vi "HW XML Rx - Write.vi"(0 "String (in)":string, 2 "Selected Channels":i32[](array[numeric]), 7 "Parameter Array":T1[](array[typedef])) -> (4 "String (out)":string)   [LabVIEW 2017]
uses:
  Controls/Database_Array.ctl
  Controls/Encoding.ctl
  <userlib>/_OpenG.lib/array/array.llb/Remove Duplicates from 1D Array (I32)__ogtk.vi
  <userlib>/_OpenG.lib/array/array.llb/Filter 1D Array with Scalar (I32)__ogtk.vi
  <userlib>/_OpenG.lib/array/array.llb/Index 1D Array Elements (Variant)__ogtk.vi
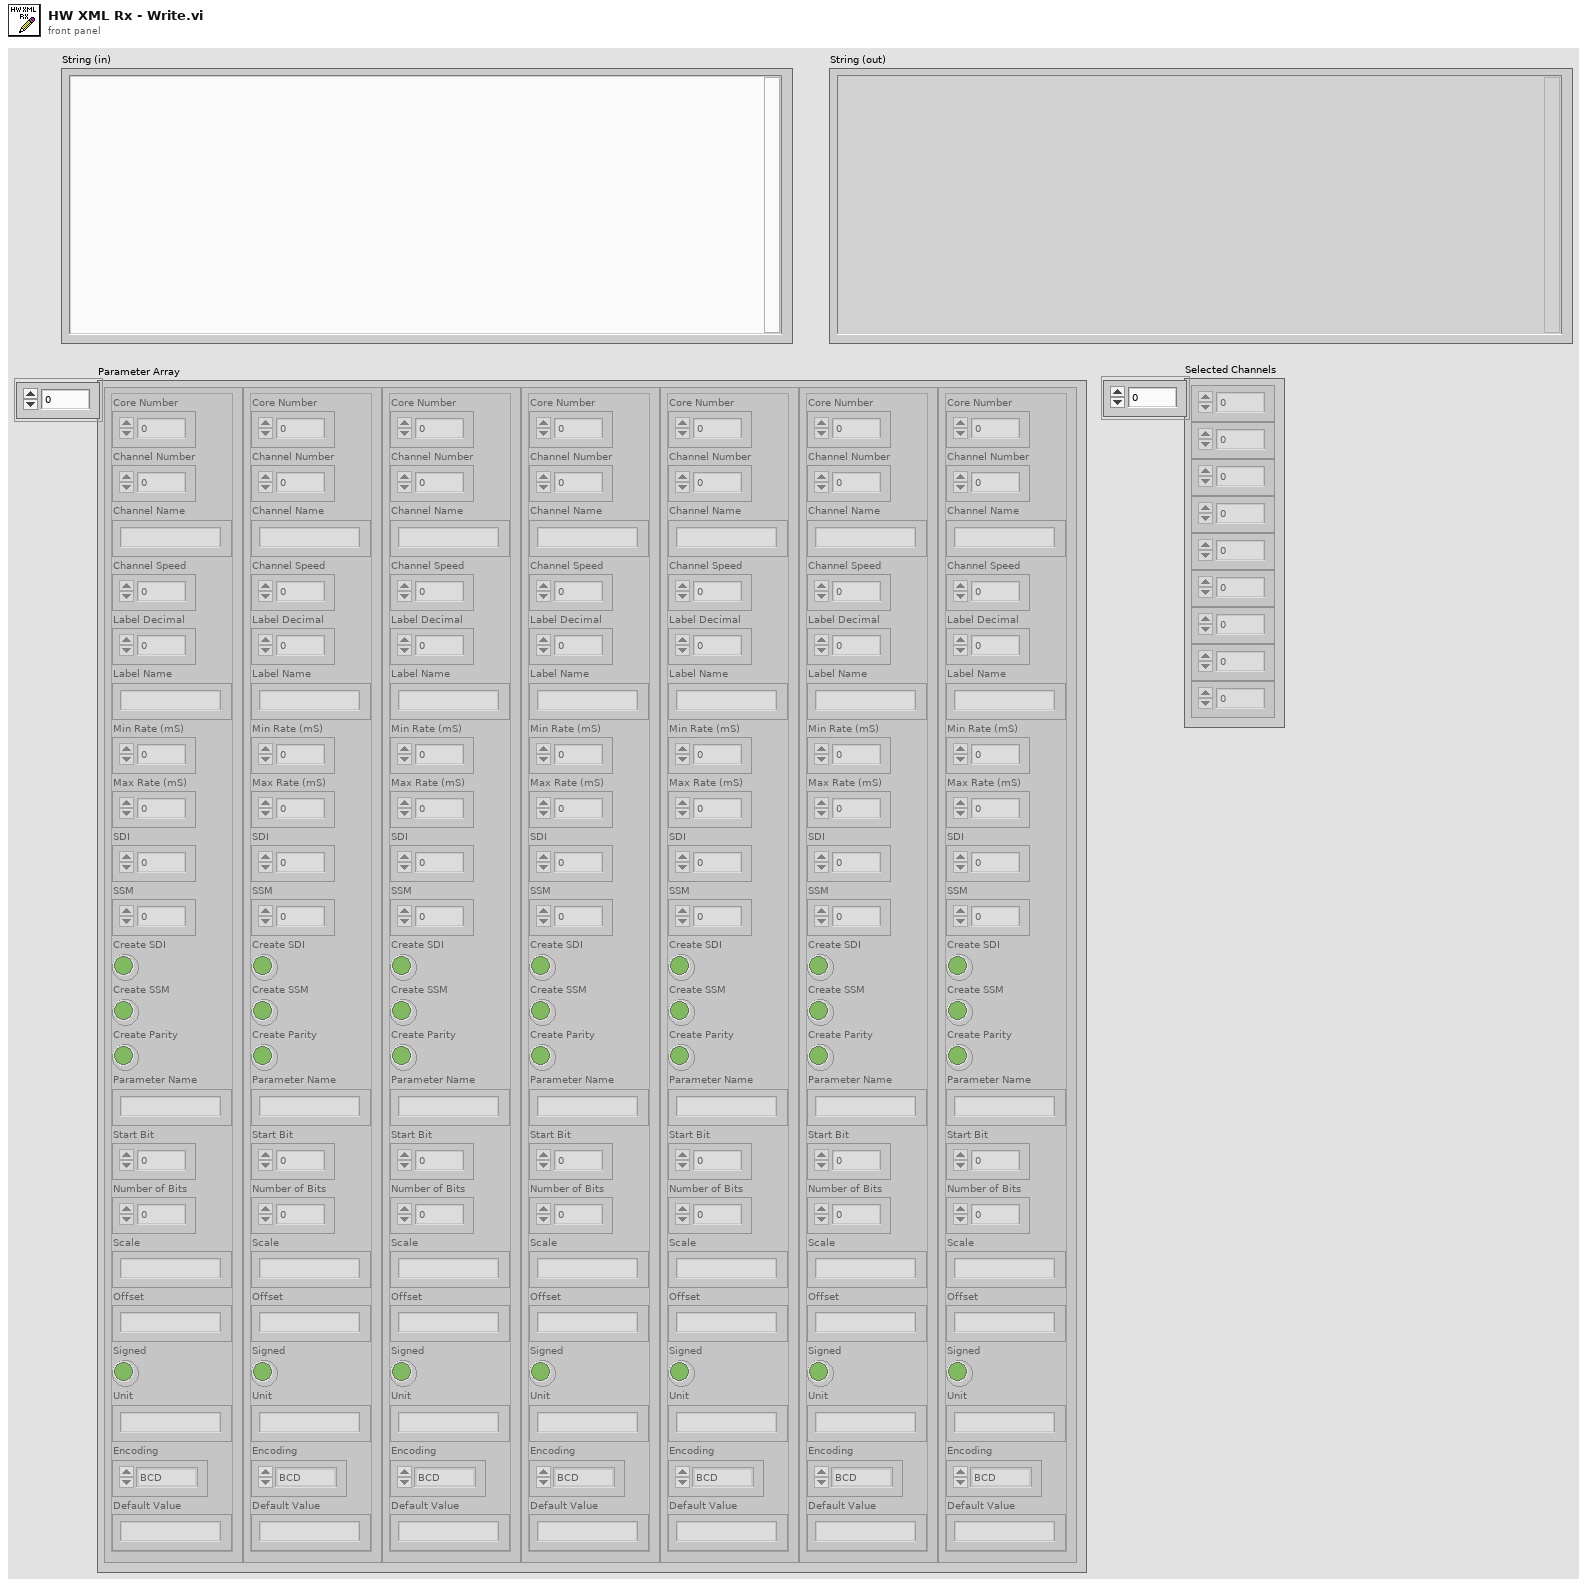
[diagram p1: front panel]
types:
  T1 = typedef "Database_Array.ctl" = cluster{"Core Number":i32, "Channel Number":i32, "Channel Name":string, "Channel Speed":i32, "Label Decimal":i32, "Label Name":string, "Min Rate (mS)":i32, "Max Rate (mS)":i32, "SDI":i32, "SSM":i32, "Create SDI":bool, "Create SSM":bool, "Create Parity":bool, "Parameter Name":string, "Start Bit":i32, "Number of Bits":i32, "Scale":string, "Offset":string, "Signed":bool, "Unit":string, "Encoding":T2, "Default Value":string}
  T2 = typedef "Encoding.ctl" = enum16{"BCD", "BNR", "Discrete"}
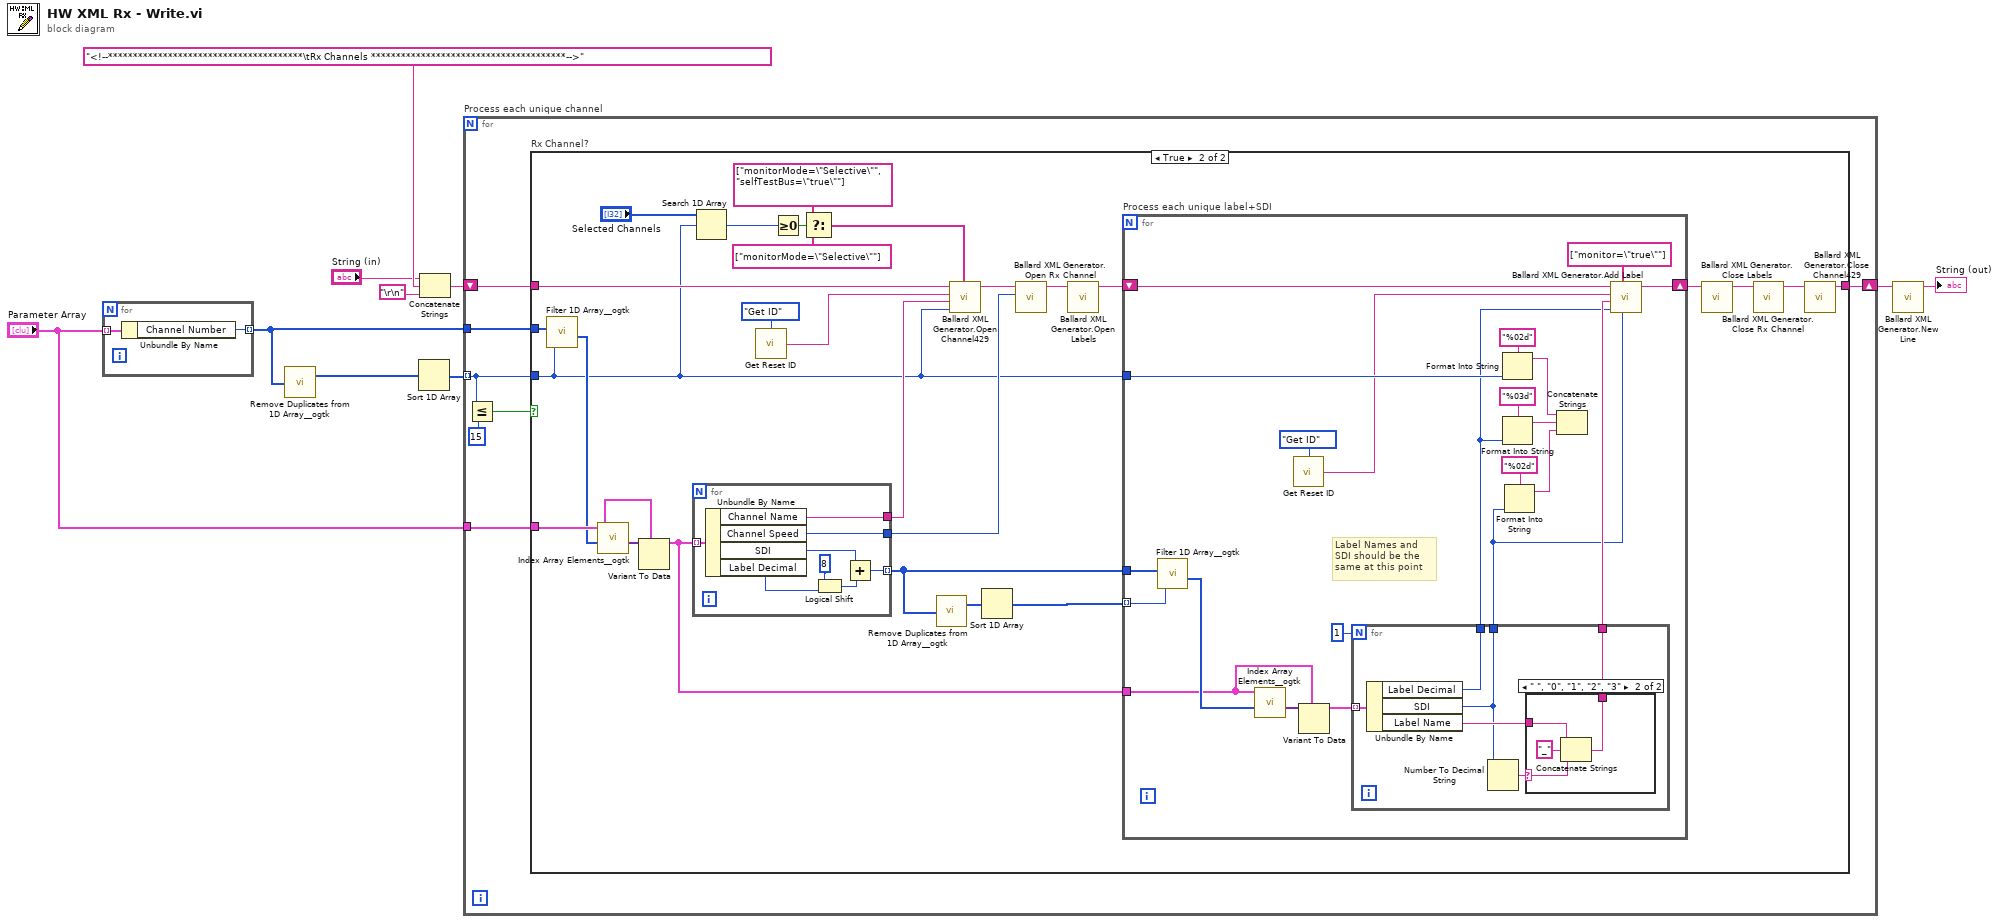
[diagram p0: block diagram]
diagram:
  n1 = for {
    tunnel: [w12] -> w3 mode=indexing
    tunnel: "Parameter Array" -> [w11] mode=indexing
    n2 = Unbundle By Name(w11) -> ("Channel Number"=w12:i32)
  }
  n3 = call-poly <userlib>:"Remove Duplicates from 1D Array__ogtk.vi"("Input Array"=w3) -> ("Output Array"=w9:i32[])  [unwired: 1 out]
  n4 = Sort 1D Array(array=w9) -> (sorted array=w10:i32[])
  n5 = Concatenate Strings("String (in)", "<!--***************************************\tRx Channels ***************************************-->", "\r\n") -> (w6:string)
  n6 = for "Process each unique channel" {
    tunnel: w10 -> [w17] mode=indexing
    shift-right: [w18] -> w1
    shift-left: w6 -> [w19]
    tunnel: w3 -> [w14]
    tunnel: "Parameter Array" -> [w13]
    n7 = Less Or Equal?(x=w17, y=15) -> (x <= y?=w16:bool)
    n8 = case "Rx Channel?" shown="True" w16 {
      tunnel: w19 -> [w20 w45]
      tunnel: [w20 w38] -> w18
      tunnel: w17 -> [_ w26]
      tunnel: w14 -> [_ w37]
      tunnel: w13 -> [_ w35]
      frame False {
      }
      frame True {
        n9 = call-poly <userlib>:"Filter 1D Array__ogtk.vi"("items to filter"=w26, "array"=w37) -> ("filtered item indices"=w33:i32[])  [unwired: 4 in, 1 out]
        n10 = call-poly <userlib>:"Index Array Elements__ogtk.vi"("indices"=w33, "array"=w35) -> ("elements"=w36:variant[])  [unwired: 9 in]
        n11 = Variant To Data(type=w35, Variant=w36) -> (data=w32:T1[])  [unwired: 1 in, 1 out]
        n12 = for {
          tunnel: w32 -> [w55] mode=indexing
          tunnel: [w54] -> w31
          tunnel: [w53] -> w30
          tunnel: [w49] -> w34 mode=indexing
          n13 = Unbundle By Name(w55) -> ("Channel Name"=w54:string, "Channel Speed"=w53:i32, "SDI"=w48:i32, "Label Decimal"=w50:i32)
          n14 = Logical Shift(y=i16 8, x=w50) -> (x << y=w52:i32)
          n15 = Add(x=w48, y=w52) -> (x+y=w49:i32)
        }
        n16 = Search 1D Array(1D array="Selected Channels", element=w26) -> (index of element=w25:i32)  [unwired: 1 in]
        n17 = call "Get Reset ID.vi"("Function"=enum16{"Get ID", "Reset ID"}."Get ID") -> ("ID"=w28:string)  [unwired: 14 in]
        n18 = Greater Or Equal To 0?(x=w25) -> (x >= 0?=w24:bool)
        n19 = Select(t=string[] ["monitorMode=\"Selective\"", "selfTestBus=\"true\""] ("other params"), s=w24, f=string[] ["monitorMode=\"Selective\""] ("other params")) -> (s? t:f=w21:string[])
        n20 = call-poly <userlib>:"Remove Duplicates from 1D Array__ogtk.vi"("Input Array"=w34) -> ("Output Array"=w47:i32[])  [unwired: 1 out]
        n21 = call "Ballard XML Generator.Open Channel429.vi"("other params"=w21, "hardware channel"=w26, "name"=w31, "id"=w28, "string in"=w45) -> ("string out"=w43:string)  [unwired: 6 in]
        n22 = Sort 1D Array(array=w47) -> (sorted array=w46:i32[])
        n23 = call "Ballard XML Generator.Open Rx Channel.vi"("speedKHz"=w30, "string in"=w43) -> ("string out"=w44:string)  [unwired: 9 in]
        n24 = call "Ballard XML Generator.Open Labels.vi"("string in"=w44) -> ("string out"=w42:string)  [unwired: 10 in]
        n25 = for "Process each unique label+SDI" {
          tunnel: w46 -> [w71] mode=indexing
          tunnel: w34 -> [w77]
          shift-right: [w74] -> w41
          shift-left: w42 -> [w75]
          tunnel: w26 -> [w70]
          tunnel: w32 -> [w65]
          # "Label Names and SDI should be the same at this point"
          n26 = call-poly <userlib>:"Filter 1D Array__ogtk.vi"("items to filter"=w71, "array"=w77) -> ("filtered item indices"=w67:i32[])  [unwired: 4 in, 1 out]
          n27 = call-poly <userlib>:"Index Array Elements__ogtk.vi"("indices"=w67, "array"=w65) -> ("elements"=w66:variant[])  [unwired: 9 in]
          n28 = call "Get Reset ID.vi"("Function"=enum16{"Get ID", "Reset ID"}."Get ID") -> ("ID"=w56:string)  [unwired: 14 in]
          n29 = Variant To Data(type=w65, Variant=w66) -> (data=w64:T1[])  [unwired: 1 in, 1 out]
          n30 = for {
            N: 1 -> [_]
            tunnel: w64 -> [w83] mode=indexing
            tunnel: [w81] -> w63
            tunnel: [w82] -> w62
            tunnel: [w78] -> w58
            n31 = Unbundle By Name(w83) -> ("Label Decimal"=w82:i32, "SDI"=w78:i32, "Label Name"=w79:string)
            n32 = Number To Decimal String(number=w78) -> (decimal integer string=w80:string)  [unwired: 1 in]
            n33 = case shown="\" \", \"0\", \"1\", \"2\", \"3\"" w80 {
              selector: w80 -> [_ w85]
              tunnel: w79 -> [w84 w88]
              tunnel: [w84 w86] -> w81
              frame "False", Default {
              }
              frame " ", "0", "1", "2", "3" {
                n34 = Concatenate Strings(w88, "_" ("string"), w85) -> (w86:string)
              }
            }
          }
          n35 = Format Into String(format string="%02d", w70) -> (resulting string=w69:string)  [unwired: 2 in, 1 out]
          n36 = Format Into String(format string="%03d", w62) -> (resulting string=w68:string)  [unwired: 2 in, 1 out]
          n37 = Format Into String(format string="%02d", w58) -> (resulting string=w59:string)  [unwired: 2 in, 1 out]
          n38 = Concatenate Strings(w69, w68, w59) -> ()  [unwired: 1 out]
          n39 = call "Ballard XML Generator.Add Label.vi"("SDI"=w58, "other params"=string[] ["monitor=\"true\""], "label decimal"=w62, "name"=w63, "id"=w56, "string in"=w75) -> ("string out"=w74:string)  [unwired: 5 in]
        }
        n40 = call "Ballard XML Generator.Close Labels.vi"("string in"=w41) -> ("string out"=w40:string)  [unwired: 10 in]
        n41 = call "Ballard XML Generator.Close Rx Channel.vi"("string in"=w40) -> ("string out"=w39:string)  [unwired: 10 in]
        n42 = call "Ballard XML Generator.Close Channel429.vi"("string in"=w39) -> ("string out"=w38:string)  [unwired: 10 in]
      }
    }
  }
  n43 = call "Ballard XML Generator.New Line.vi"("string in"=w1) -> ("string out"=→"String (out)":string)  [unwired: 10 in]
